vi "test4.vi"() -> ()   [LabVIEW 2014]
panel:
  out "Temps écoulé":dbl(knob) scale=0.0..60.0
  in  "Durée du programme":dbl
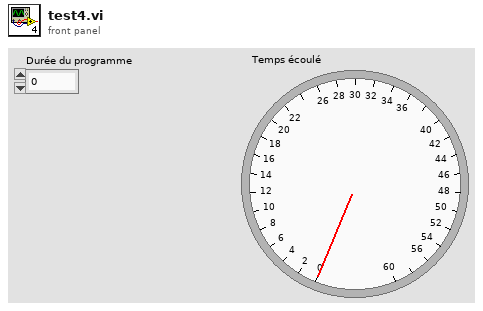
[diagram p1: front panel]
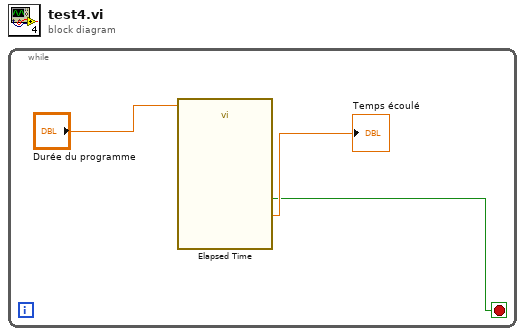
[diagram p0: block diagram]
diagram:
  n1 = while {
    stop <- w1 stop-if-true
    n2 = call "Elapsed Time"("Time Target (s)"="Durée du programme") -> ("Elapsed Time (s)"=→"Temps écoulé":dbl, "Time has Elapsed"=w1:bool)  [unwired: 11 in, 6 out]
  }
